vi "Classify Instrument VIs.vi"(0 "InstrContaining":path[][](array[path]), 5 "DestinationDirectory":path[](array[path]), 11 "error in (no error)":errorcluster) -> (4 "InstrContainingVI[]":path[][](array[path]), 15 "error out":errorcluster)   [LabVIEW 2021, in "Multiple Migrator.lvlib"]
uses:
  Multiple Migrator.lvlib
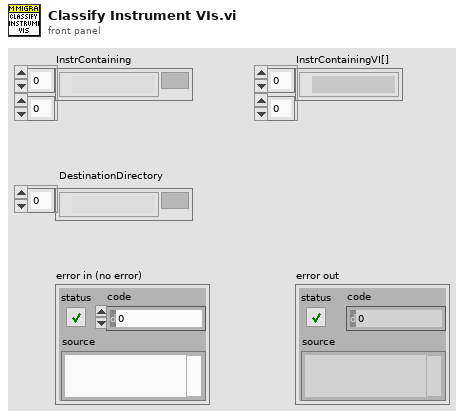
[diagram p1: front panel]
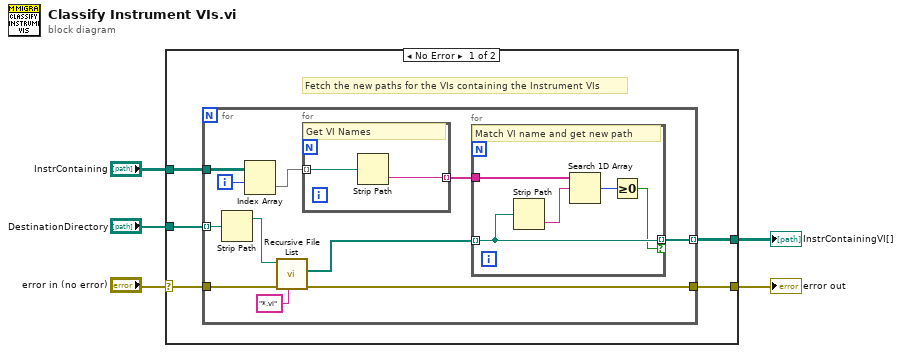
[diagram p0: block diagram]
diagram:
  n1 = case shown="No Error" "error in (no error)" {
    selector: "error in (no error)" -> [w9 w29]
    tunnel: [w7 w29] -> w5
    tunnel: [w10 _] -> w4
    tunnel: "InstrContaining" -> [w8 _]
    tunnel: "DestinationDirectory" -> [w6 _]
    frame No Error {
      # "Fetch the new paths for the VIs containing the Instrument VIs"
      n2 = for {
        tunnel: [w21] -> w10 mode=indexing
        tunnel: w8 -> [w19]
        tunnel: w6 -> [w12] mode=indexing
        tunnel: [w15] -> w7
        tunnel: w9 -> [w14]
        i -> [w18]
        n3 = Strip Path(path=w12) -> (stripped path=w11:path)  [unwired: 1 out]
        n4 = Index Array(array=w19, index (row)=w18) -> (element=w17:path[])  [unwired: 1 in]
        n5 = call <vilib>:"Recursive File List.vi"("pattern"="*.vi", "error in (no error)"=w14, "Folder Path"=w11) -> ("error out"=w15:errorcluster, "All Files in Dir"=w13:path[])  [unwired: 4 in, 3 out]
        n6 = for {
          tunnel: w17 -> [w23] mode=indexing
          tunnel: [w22] -> w20 mode=indexing
          # "Get VI Names"
          n7 = Strip Path(path=w23) -> (name=w22:string)  [unwired: 1 out]
        }
        n8 = for {
          tunnel: w13 -> [w25] mode=indexing
          tunnel: w20 -> [w28]
          tunnel: [w25] -> w21 mode=indexing if=w24
          # "Match VI name and get new path"
          n9 = Strip Path(path=w25) -> (name=w27:string)  [unwired: 1 out]
          n10 = Search 1D Array(1D array=w28, element=w27) -> (index of element=w26:i32)  [unwired: 1 in]
          n11 = Greater Or Equal To 0?(x=w26) -> (x >= 0?=w24:bool)
        }
      }
    }
    frame Error {
    }
  }
  "error out" <- w5
  "InstrContainingVI[]" <- w4
